vi "VI-File-Explorer.vi"() -> ()   [LabVIEW 2021, in "vi_lib.lvlib"]
uses:
  vi_lib.lvlib
  clLabview/clLabview.lvclass
  clFile/clFile.lvclass
panel:
  out "concatenated string":string
  in  "new VI-Lib Password":string
  in  "Update LV-Lib Password":bool
  out "File is protected?":bool=TRUE
  out "LV-Lib password (Hex)":string
  out "Icon":picture
  out "busy (*)":bool
  out "Salt (Hex)":string
  out "MD5-Hash 2 (Hex)":string
  out "MD5-Hash 1 (Hex)":string
  out "saving done":bool
  in  "save":bool
  in  "Open":bool
  in  "stop":bool
  out "flags":i32 step=1
  out "stage":u8(ring) items=["development", "alpha", "beta", "release"]
  out "build":u8 step=1
  out "bugfix":u8 step=1
  out "minor":u8 max=99 step=1
  out "major":u8=3 min=1 max=99 step=1
  out "version info":string
  out "version text":string
  in  "save to":path=path "D:/labview/file_in_(free).vi"
  in  "new File Password":string
  in  "open from":path=path "D:/labview/file.vi"
  out "MD5 password (Hex)":string
  # "MD5 password (Hex)\nMD5-Hash 1 (Hex)\nMD5-Hash 2 (Hex) for LV-Version >= 8\nLV-Lib password (Hex)"
  # "File password [BDPW]"
  # "for LV-Version >= 8"
  # "for LV-Version >= 12"
  # "(*) This is a \"brute force\" version to calc the password Salt, \n      so it might take up to 30sec."
  # "File propertys [LVSR]"
  # "File version [vers]"
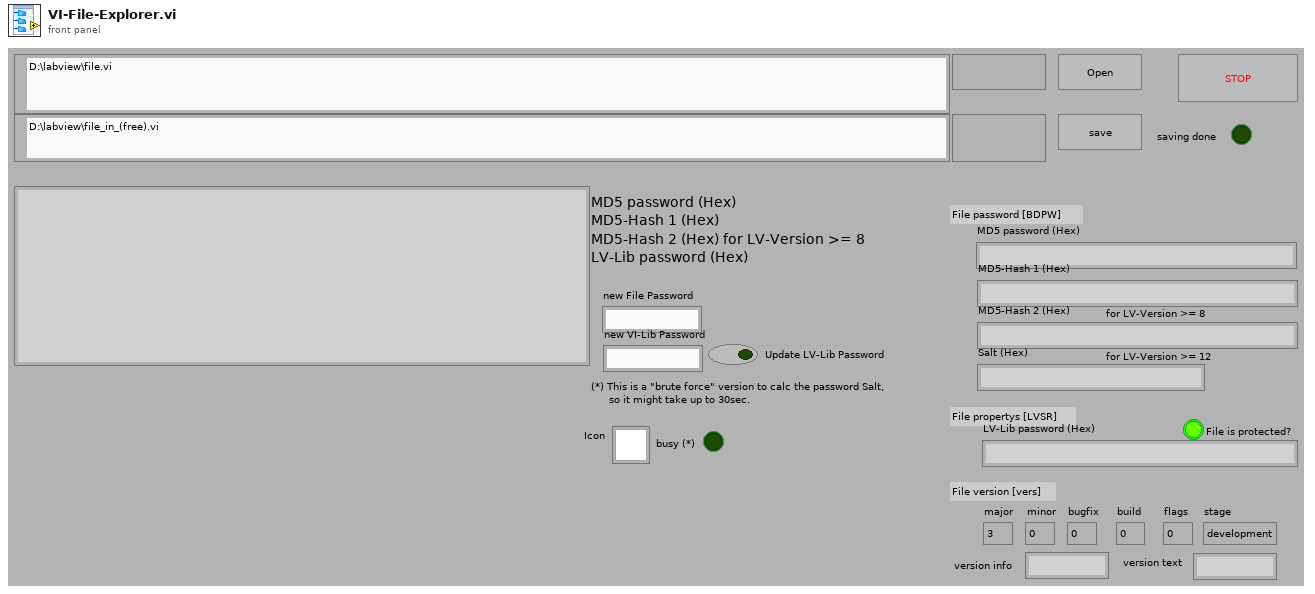
[diagram p1: front panel]
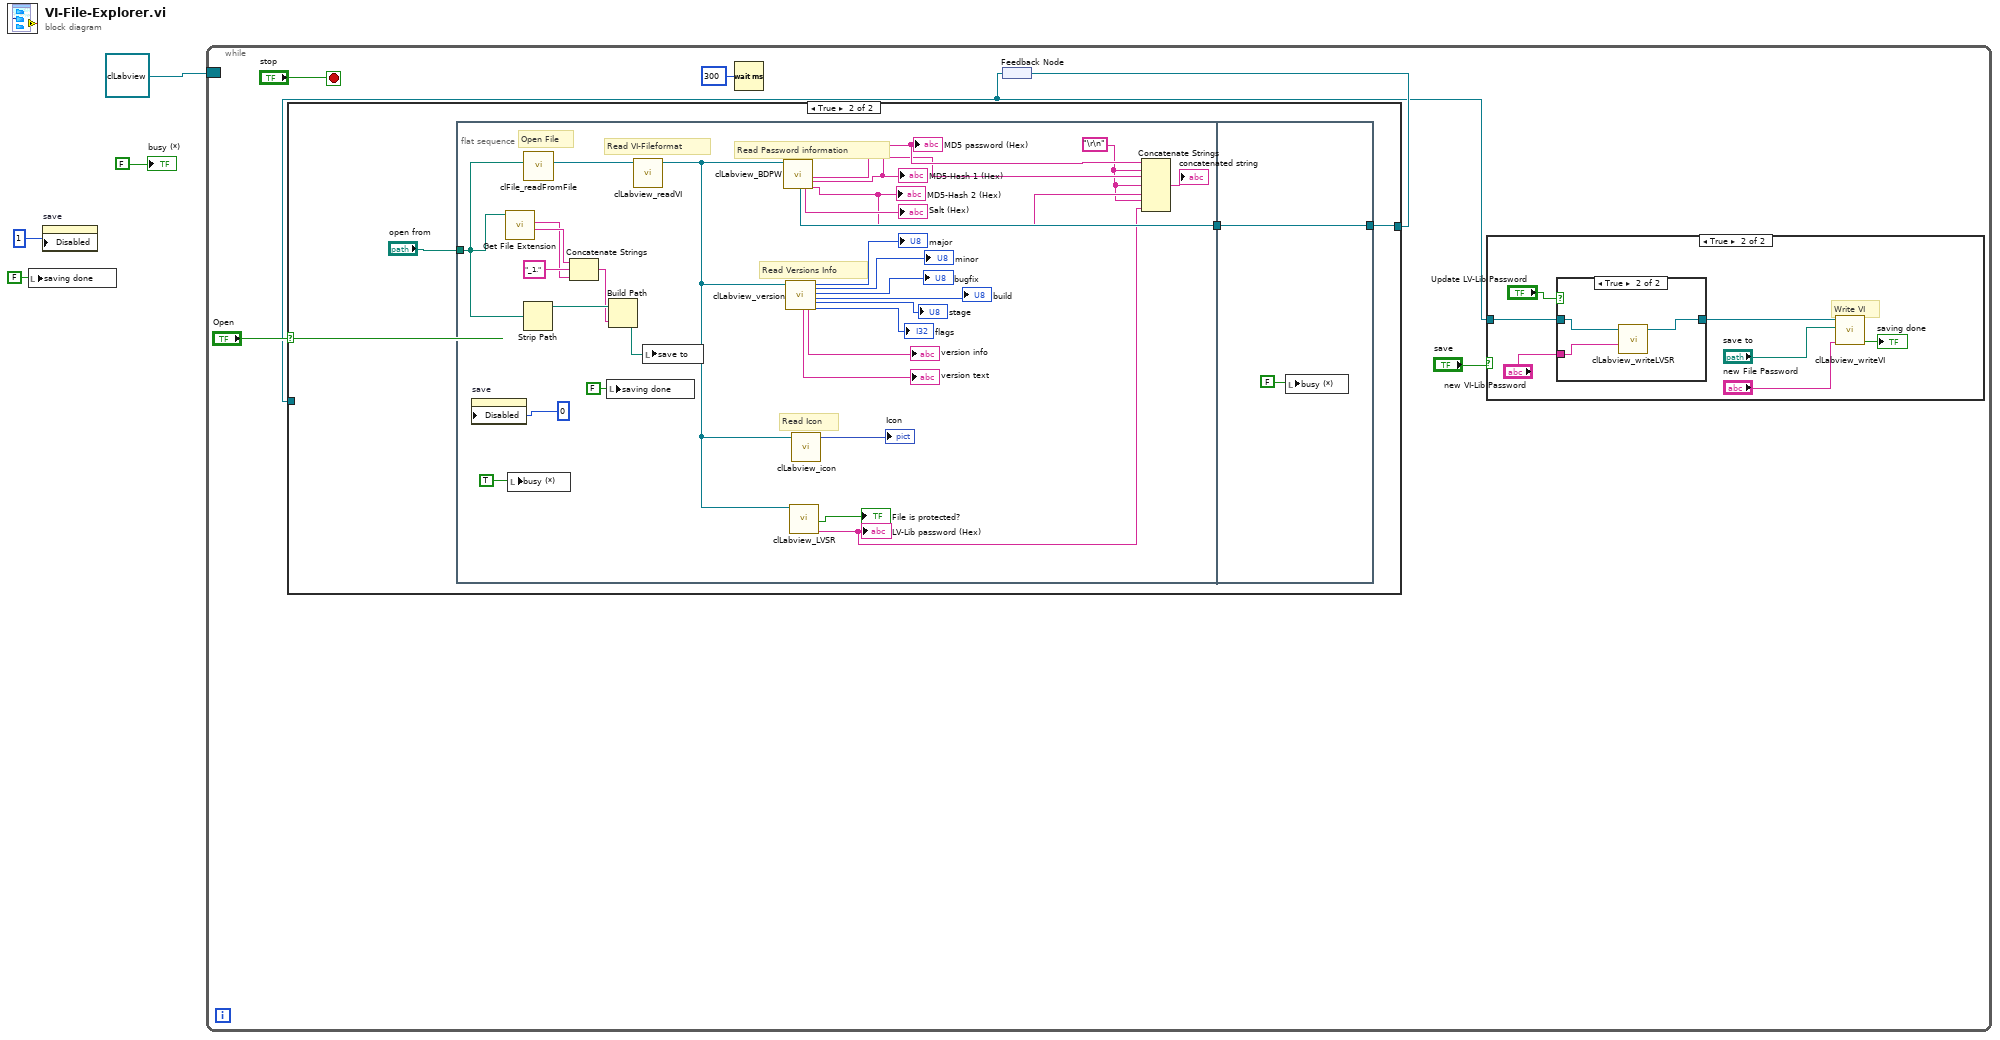
[diagram p0: block diagram]
diagram:
  n1 = local write "saving done"(FALSE ("saving done")) -> ()
  n2 = property on="save" class="Bool"("Disabled"=u8 1) -> ()  [unwired: 2 in, 2 out]
  n3 = while {
    border: refnum<class "clLabview.lvclass"> refnum ("vi_lib.lvlib:clLabview.lvclass 2") -> [_]
    stop <- "stop" stop-if-true
    n4 = Wait (ms)(milliseconds to wait=u32 300) -> ()  [unwired: 1 out]
    n5 = feedback #1() -> (w6:refnum<class "clLabview.lvclass">)
    n6 = case shown="True" "Open" {
      tunnel: [w22 w25] -> w8
      tunnel: w6 -> [w22 _]
      frame False {
      }
      frame True {
        n7 = flat-sequence {
          tunnel: [w44] -> w24
          tunnel: "open from" -> [w26]
          tunnel: [w57] -> w25
          tunnel: w24 -> [w57]
          frame #0 {
            w29 = "\r\n"
            # "Read Icon"
            # "Read Versions Info"
            # "Read Password information"
            # "Read VI-Fileformat"
            # "Open File"
            n8 = property on="save" class="Bool"("Disabled"=u8 0) -> ()  [unwired: 2 in, 2 out]
            n9 = call <vilib>:"Get File Extension.vi"("file"=w26) -> ("filename without extension"=w37:string, "lowercase file extension"=w35:string)  [unwired: 6 in, 3 out]
            n10 = local write "busy (*)"(TRUE ("busy")) -> ()
            n11 = Strip Path(path=w26) -> (stripped path=w39:path)  [unwired: 1 out]
            n12 = call "clFile_readFromFile.vi"("file (use dialog)"=w26) -> ("clFileReader.lvclass"=w55:refnum<class "clFileReader.lvclass">)  [unwired: 1 in, 9 out]
            n13 = Concatenate Strings(w37, "_1." ("string"), w35) -> (w34:string)
            n14 = local write "saving done"(FALSE ("saving done")) -> ()
            n15 = Build Path(base path=w39, name or relative path=w34) -> (appended path=w38:path)
            n16 = call "clLabview_readVI.vi"("vi_lib.lvlib:clFileReader.lvclass"=w55) -> ("vi_lib.lvlib:clLabview.lvclass 2"=w41:refnum<class "clLabview.lvclass">)  [unwired: 10 out]
            n17 = local write "save to"(w38) -> ()
            n18 = call "clLabview_BDPW.vi"("vi_lib.lvlib:clLabview.lvclass"=w41) -> ("vi_lib.lvlib:clLabview.lvclass [Out]"=w44:refnum<class "clLabview.lvclass">, "Salt (Hex)"=→"Salt (Hex)":string, "MD5 password (Hex)"=w33:string, "MD5-Hash 1  (Hex)"=w32:string, "MD5-Hash 2  (Hex)"=w31:string)  [unwired: 14 out]
            "MD5 password (Hex)" <- w33
            "MD5-Hash 2 (Hex)" <- w31
            "MD5-Hash 1 (Hex)" <- w32
            n19 = call "clLabview_version.vi"("vi_lib.lvlib:clLabview.lvclass"=w41) -> ("version_text"=→"version text":string, "version_info"=→"version info":string, "major"=→"major":u8, "minor"=→"minor":u8, "bugfix"=→"bugfix":u8, "build"=→"build":u8, "stage"=→"stage":u8, "flags"=→"flags":i32)  [unwired: 11 out]
            n20 = call "clLabview_LVSR.vi"("vi_lib.lvlib:clLabview.lvclass"=w41) -> ("File is protected?"=→"File is protected?":bool, "MD5 lib Password (Hex)"=w28:string)  [unwired: 17 out]
            "LV-Lib password (Hex)" <- w28
            n21 = call "clLabview_icon.vi"("vi_lib.lvlib:clLabview.lvclass"=w41) -> ("Icon"=→"Icon":picture)  [unwired: 10 out]
            n22 = Concatenate Strings(w33, w29, w32, w29, w31, w29, w28) -> (→"concatenated string":string)
          }
          frame #1 {
            n23 = local write "busy (*)"(FALSE ("busy")) -> ()
          }
        }
      }
    }
    n24 = feedback-in #1(w8) -> ()
    n25 = case shown="True" "save" {
      tunnel: w6 -> [_ w13]
      frame False {
      }
      frame True {
        # "Write VI"
        n26 = case shown="True" "Update LV-Lib Password" {
          tunnel: w13 -> [w18 w21]
          tunnel: [w18 w20] -> w14
          tunnel: "new VI-Lib Password" -> [_ w19]
          frame False {
          }
          frame True {
            n27 = call "clLabview_writeLVSR.vi"("vi_lib.lvlib:clLabview.lvclass"=w21, "new lib Password"=w19) -> ("vi_lib.lvlib:clLabview.lvclass [Out]"=w20:refnum<class "clLabview.lvclass">)  [unwired: 8 out]
          }
        }
        n28 = call "clLabview_writeVI.vi"("vi_lib.lvlib:clLabview.lvclass"=w14, "filename (use dialog)"="save to", "new Password"="new File Password") -> ("no Error"=→"saving done":bool)  [unwired: 7 out]
      }
    }
  }
  "busy (*)" <- FALSE ("busy")
